vi "DPO_7K_Get_Array_Scales.vi"(8 "Error in":errorcluster, 10 "Channel":u16(ring) items=["Channel 1", "Channel 2", "Channel 3", "Channel 4", "Math 1", "Math 2", "Math 3", "Math 4", "Reference 1", "Reference 2", "Reference 3", "Reference 4"], 11 "VISA resource name in":refnum<visa-resource-name>) -> (0 "Error out":errorcluster, 2 "Scale Array":dbl[](array[numeric]), 3 "VISA resource name out":refnum<visa-resource-name>)   [LabVIEW 2020]
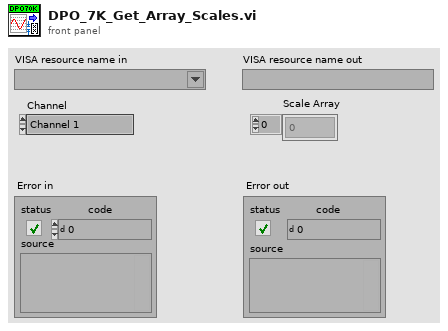
[diagram p1: front panel]
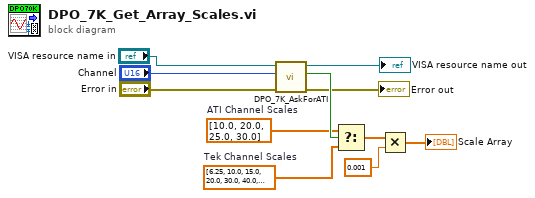
[diagram p0: block diagram]
diagram:
  w8 = dbl[] [10.0, 20.0, 25.0, 30.0]  # ATI Channel Scales
  w7 = dbl[] [6.25, 10.0, 15.0, 20.0, 30.0, 40.0, 50.0, 60.0, 70.0, 80.0, 90.0, 100.0, 110.0, 120.0, 200.0, 300.0, 400.0, 500.0, 600.0]  # Tek Channel Scales
  n1 = call "DPO_7K_AskForATI.vi"("Error In"="Error in", "Channel"="Channel", "VISA resource name in"="VISA resource name in") -> ("Error Out"=→"Error out":errorcluster, "ATI?"=w9:bool, "VISA resource name out"=→"VISA resource name out":refnum<visa-resource-name>)  [unwired: 6 in]
  n2 = Select(t=w8, s=w9, f=w7) -> (s? t:f=w3:dbl[])
  n3 = Multiply(x=w3, y=0.001) -> (x*y=→"Scale Array":dbl[])
